vi "Plot attributes load.vi"(8 "error in (no error)":errorcluster, 9 "attributes":T1, 10 "Active Plot":u32, 11 "Plot":refnum<vi>) -> (0 "error out":errorcluster, 3 "plot":refnum<vi>)   [LabVIEW 2021, in "RocketPlot.lvlib"]
uses:
  RocketPlot.lvlib
  TypeDefs/plot attributes V2.ctl
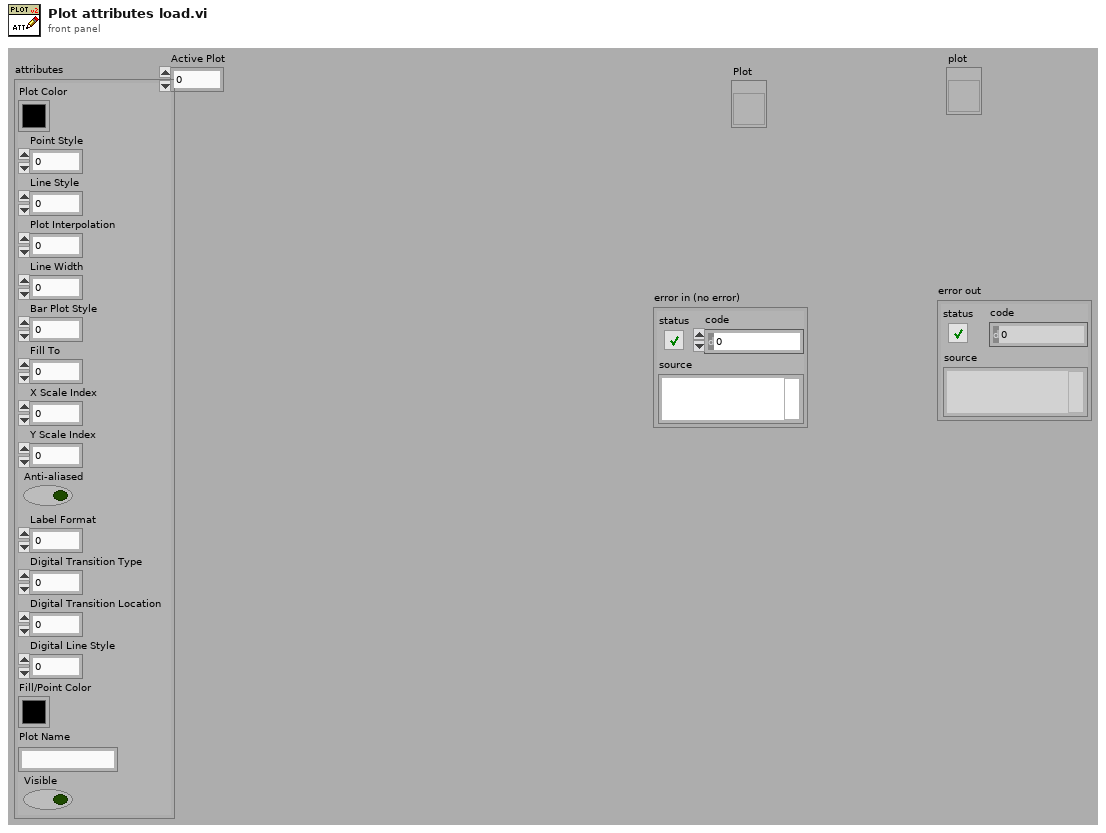
[diagram p1: front panel]
types:
  T1 = typedef "RocketPlot.lvlib/plot attributes V2.ctl" = cluster{"Plot Color":u32, "Point Style":u8, "Line Style":u8, "Plot Interpolation":u8, "Line Width":u8, "Bar Plot Style":u8, "Fill To":i16, "X Scale Index":u32, "Y Scale Index":u32, "Anti-aliased":bool, "Label Format":u8, "Digital Transition Type":u8, "Digital Transition Location":u8, "Digital Line Style":u8, "Fill/Point Color":u32, "Plot Name":string, "Visible":bool}
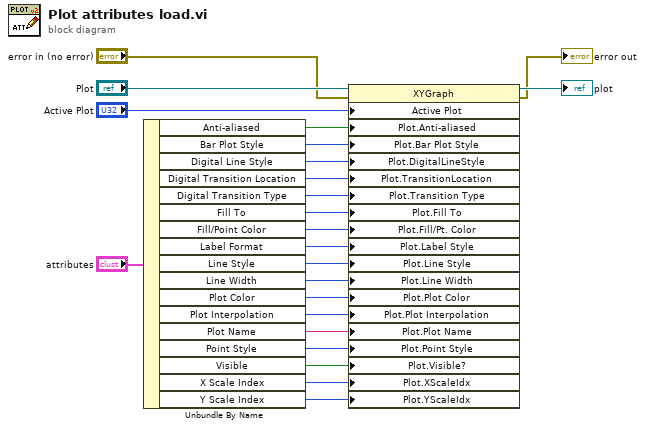
[diagram p0: block diagram]
diagram:
  n1 = Unbundle By Name("attributes") -> ("Anti-aliased"=w22:bool, "Bar Plot Style"=w21:u8, "Digital Line Style"=w20:u8, "Digital Transition Location"=w19:u8, "Digital Transition Type"=w18:u8, "Fill To"=w17:i16, "Fill/Point Color"=w16:u32, "Label Format"=w15:u8, "Line Style"=w14:u8, "Line Width"=w13:u8, "Plot Color"=w12:u32, "Plot Interpolation"=w11:u8, "Plot Name"=w10:string, "Point Style"=w9:u8, "Visible"=w8:bool, "X Scale Index"=w7:u32, "Y Scale Index"=w6:u32)
  n2 = property class="XYGraph"(reference="Plot", error in="error in (no error)", "Active Plot"="Active Plot", "Plot.Anti-aliased"=w22, "Plot.Bar Plot Style"=w21, "Plot.DigitalLineStyle"=w20, "Plot.TransitionLocation"=w19, "Plot.Transition Type"=w18, "Plot.Fill To"=w17, "Plot.Fill/Pt. Color"=w16, "Plot.Label Style"=w15, "Plot.Line Style"=w14, "Plot.Line Width"=w13, "Plot.Plot Color"=w12, "Plot.Plot Interpolation"=w11, "Plot.Plot Name"=w10, "Plot.Point Style"=w9, "Plot.Visible?"=w8, "Plot.XScaleIdx"=w7, "Plot.YScaleIdx"=w6) -> (reference out=→"plot":refnum<vi>, error out=→"error out":errorcluster)
